vi "BME_DG_ReadParameterFile_V2.vi"(8 "error in (no error)":errorcluster, 11 "Path":path=path "C:/Dokumente und Einstellungen/A2.5/Desktop/POLARIS BME DG/ParameterFiles/20120327 mit StandAloneAppl von 20120323.g0y") -> (0 "error out":errorcluster, 1 "Slave or Master":T8[](array[typedef]), 3 "#DGs":i32, 4 "CalibrateTiming":u32, 5 "CalibrationLevel":u32)   [LabVIEW 2009, in "POLARIS BME DG.lvlib"]
uses:
  POLARIS BME DG.lvlib
  BME_DG_MasterOrSlave.ctl
  Typedefs For ReadParameters()/BME_DG_BME_State.ctl
  Typedefs For ReadParameters()/BME_DG_DelayChannelData.ctl
  Typedefs For ReadParameters()/BME_DG_State_V2.ctl
  Typedefs For ReadParameters()/BME_DG_BME_Control_V2.ctl
  Typedefs For ReadParameters()/BME_DG_DelayChannelData_V2.ctl
  Typedefs For ReadParameters()/BME_DG_DelayTriggerData_V2.ctl
  BME DLL/DelayGenerator.dll
panel:
  out "DGS":T5
  in  "Cluster":T5
  out "State":T6
  in  "p_CalibrationLevel":u32
  in  "p_CalibrateTiming":u32
  in  "#DG in":i32
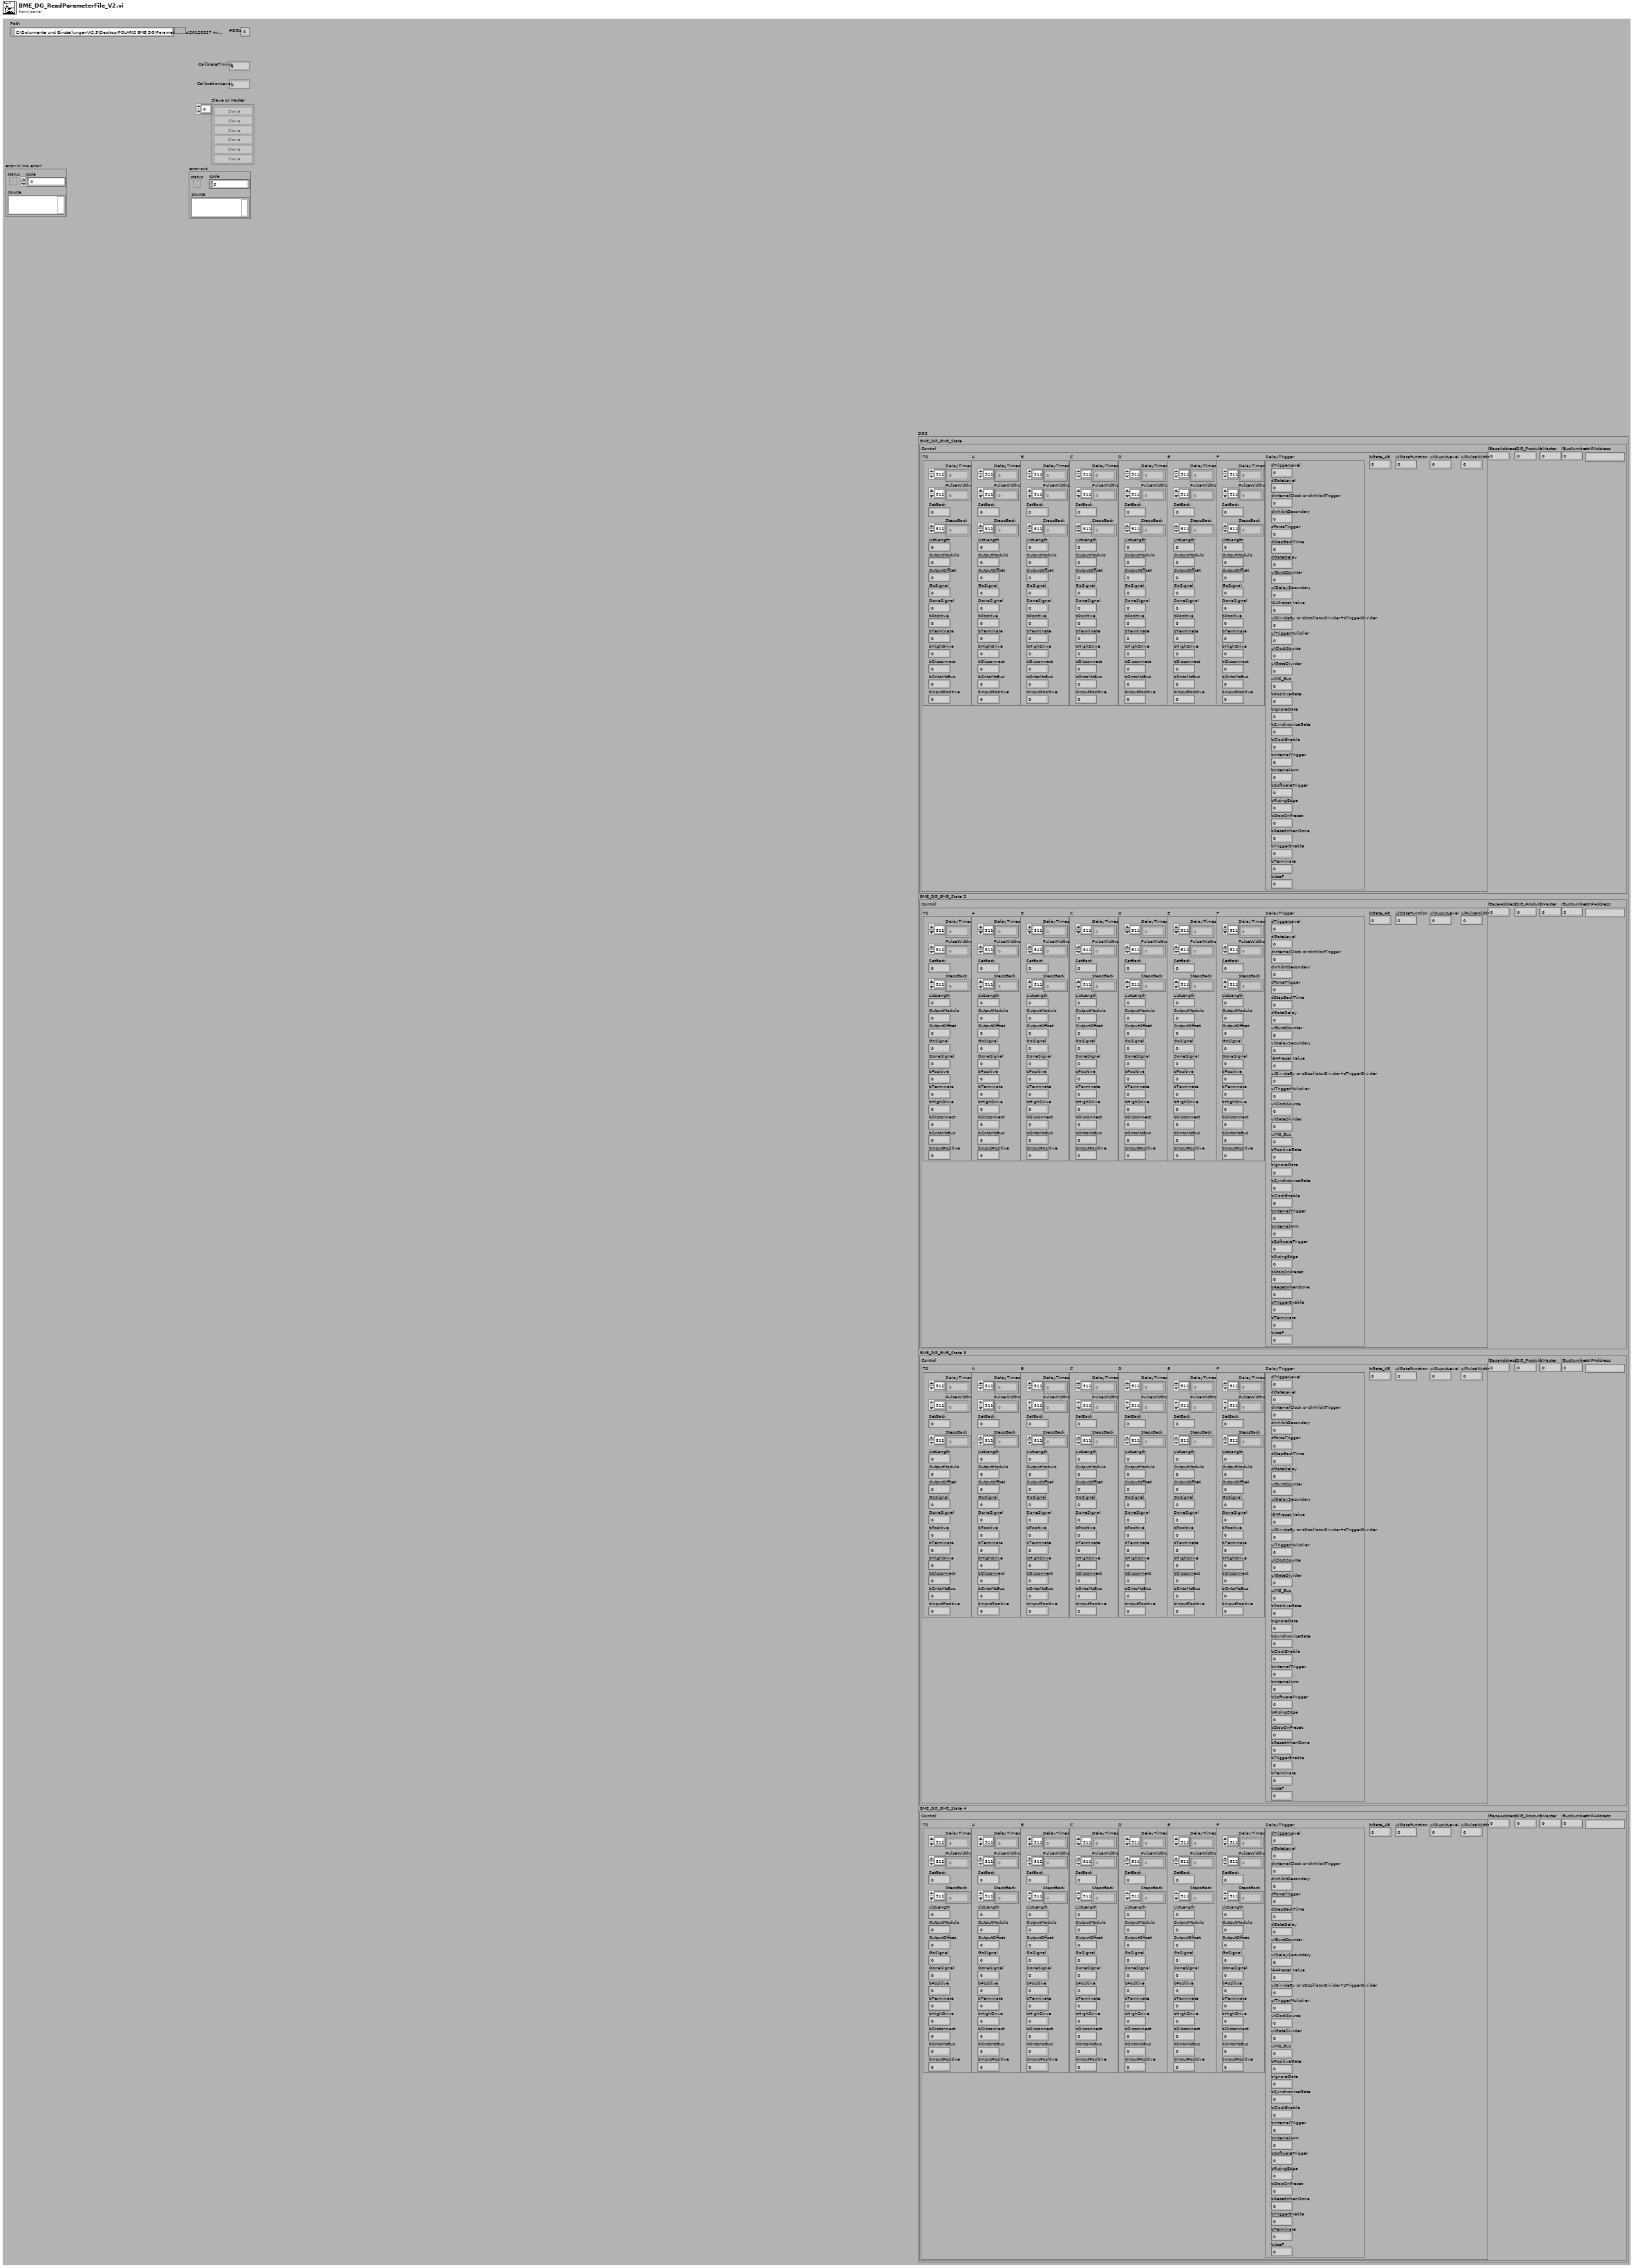
[diagram p1: front panel]
types:
  T1 = typedef "POLARIS BME DG.lvlib/BME_DG_State_V2.ctl" = cluster{"Control":T2, "lBaseAddress":i32, "lDG_Produkt":i32, "bMaster":u32, "lBusNumber":i32, "strIPAddress":string}
  T2 = typedef "POLARIS BME DG.lvlib/BME_DG_BME_Control_V2.ctl" = cluster{"T0":T3, "A":T3, "B":T3, "C":T3, "D":T3, "E":T3, "F":T3, "DelayTrigger":T4, "bGate_AB":u32, "ulGateFunction":u32, "ulOuputLevel":u32, "ulPulseWidth":u32}
  T3 = typedef "POLARIS BME DG.lvlib/BME_DG_DelayChannelData_V2.ctl" = cluster{"DelayTimes":dbl[], "PulseWidths":dbl[], "SetBack":dbl, "StepsBack":u32[], "ListLength":i32, "OutputModulo":u32, "OutputOffset":u32, "GoSignal":u32, "DoneSignal":u32, "bPositive":u32, "bTerminate":u32, "bHighDrive":u32, "bDisconnect":u32, "bOntoMsBus":u32, "bInputPositive":u32}
  T4 = typedef "POLARIS BME DG.lvlib/BME_DG_DelayTriggerData_V2.ctl" = cluster{"dTriggerLevel":dbl, "dGateLevel":dbl, "dInternalClock or dInhibitTrigger":dbl, "dInhibitSecondary":dbl, "dForceTrigger":dbl, "dStepBackTime":dbl, "dGateDelay":dbl, "ulBurstCounter":u32, "ulDelaySecundary":u32, "l64Preset Value":i64, "ulDivideBy or sOscillatorDivider+sTriggerDivider":u32, "ulTriggerMuliplier":u32, "ulClockSource":u32, "ulGateDivider":u32, "ulMS_Bus":u32, "bPositiveGate":u32, "bIgnoreGate":u32, "bSynchronizeGate":u32, "bClockEnable":u32, "bInternalTrigger":u32, "bInternalArm":u32, "bSoftwareTrigger":u32, "bRisingEdge":u32, "bStopOnPreset":u32, "bResetWhenDone":u32, "bTriggerEnable":u32, "bTerminate":u32, "bUseF":u32}
  T5 = cluster{"BME_DG_BME_State":T1, "BME_DG_BME_State 2":T1, "BME_DG_BME_State 3":T1, "BME_DG_BME_State 4":T1}
  T6 = typedef "POLARIS BME DG.lvlib/BME_DG_BME_State.ctl" = cluster{"T0":T7, "A":T7, "B":T7, "DT":cluster{"dTriggerLevel":dbl, "dInternalClock or dInhibitTrigger":dbl, "dForceTrigger":dbl, "ulPresetValue":u32, "ulDivideBy or sOscillatorDivider+sTriggerDivider":u32, "ulClockSource":u32, "ulGateDivider":u32, "ulMS_Bus":u32, "bPositiveGate":u32, "bIgnoreGate":u32, "bSynchronizeGate":u32, "bClockEnable":u32, "bInternalTrigger":u32, "bInternalArm":u32, "bSoftwareTrigger":u32, "bRisingEdge":u32, "bStopOnPreset":u32, "bResetWhenDone":u32, "bTriggerEnable":u32, "bTerminate":u32, "bReserve":u32}, "bGate_AB":u32, "ulGateFunction":u32, "ulOuputLevel":u32, "ulDG_Product":u32, "ulPulseWidth":u32, "fill int 1":i32, "fill int 2":i32, "fill int 3":i32, "fill int 4":i32, "fill int 5":i32}
  T7 = typedef "POLARIS BME DG.lvlib/BME_DG_DelayChannelData.ctl" = cluster{"FireFirst":dbl, "SetBack":dbl, "FireSecond":dbl, "OutputModulo":u32, "OutputOffset":u32, "GoSignal":u32, "DoneSignal":u32, "bPositive":u32, "bTerminate":u32, "bHighDrive":u32, "bReserve":u32}
  T8 = typedef "POLARIS BME DG.lvlib/BME_DG_MasterOrSlave.ctl" = enum16{"Unknown", "Master", "Slave"}
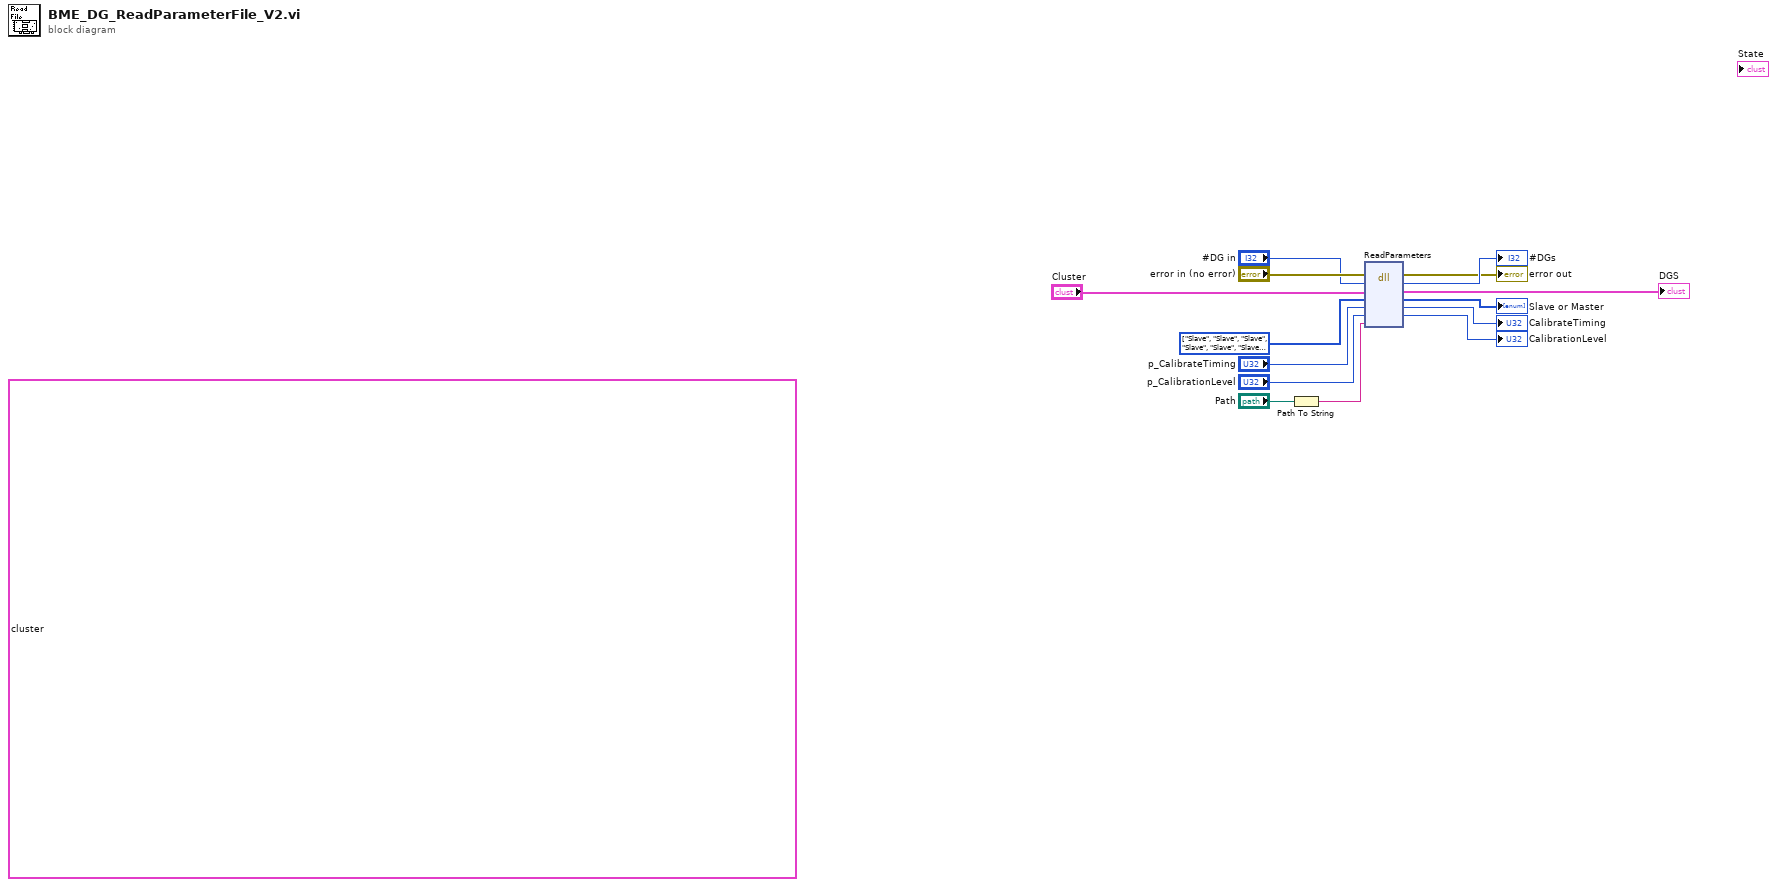
[diagram p0: block diagram]
diagram:
  (unwired) cluster{"BME_DG_BME_State":T1} data[72348B]
  w3 = T8[] [enum."Slave", enum."Slave", enum."Slave", enum."Slave", enum."Slave", enum."Slave", enum."Slave", enum."Slave", enum."Slave", enum."Slave", enum."Slave", enum."Slave", enum."Slave", enum."Slave", enum."Slave", enum."Slave", enum."Slave", enum."Slave", enum."Slave", enum."Slave", enum."Slave", enum."Slave", enum."Slave", enum."Slave", enum."Slave", enum."Slave", enum."Slave", enum."Slave", enum."Slave", enum."Slave", enum."Slave", enum."Slave", enum."Slave", enum."Slave", enum."Slave", enum."Slave", enum."Slave", enum."Slave", enum."Slave", enum."Slave", enum."Slave", enum."Slave", enum."Slave", enum."Slave", enum."Slave", enum."Slave", enum."Slave", enum."Slave", enum."Slave", enum."Slave", enum."Unknown"] items=["Unknown", "Master", "Slave"]
  n1 = Path To String(path="Path") -> (string=w10:string)
  n2 = dll-call lib="C:/CS Framework/LVSCC/LV2009/GPL/Projects/cs-framework/CSClass/CSPOLARIS/POLARIS BME DG/BME DLL/DelayGenerator.dll" fn="ReadParameters" label="Activate_DG_BME"(error in="error in (no error)", "#DG"="#DG in", "DGS"="Cluster", "module"=w3, "CalibrateTiming"="p_CalibrateTiming", "CalibrationLevel"="p_CalibrationLevel", "FileName"=w10) -> (error out=→"error out":errorcluster, "#DG"=→"#DGs":i32, "DGS"=→"DGS":T5, "module"=→"Slave or Master":i32[], "CalibrateTiming"=→"CalibrateTiming":u32, "CalibrationLevel"=→"CalibrationLevel":u32)  [unwired: 2 in, 1 out]
